vi "Download OD Values.vi"(8 "error in":errorcluster, 10 "Values":T1(array[cluster]) {"Multiplexer"."Index" format="%.0x"}, 11 "Interactor in":refnum<class "Interactor.lvclass">) -> (0 "error out":errorcluster, 3 "Interactor out":refnum<class "Interactor.lvclass">)   [LabVIEW 2024, in "Interactor.lvlib" / "Interactor.lvclass"]
uses:
  Interactor.lvclass
  Interactor.lvclass/Interactor.ctl
  CANopen Master/CANopen Master.lvclass
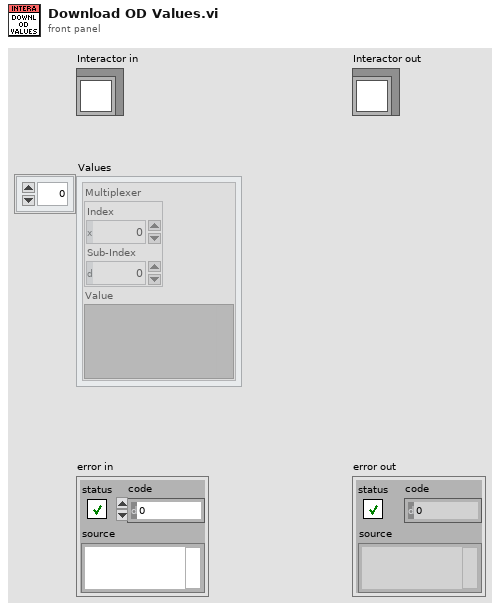
[diagram p1: front panel]
types:
  T1 = cluster{"Multiplexer":cluster{"Index":u16, "Sub-Index":i16}, "Value":variant}[]
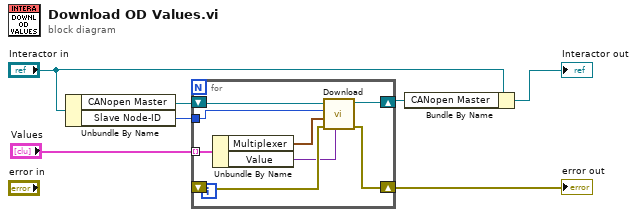
[diagram p0: block diagram]
diagram:
  n1 = Unbundle By Name("Interactor in") -> ("CANopen Master"=w5:refnum<class "CANopen Master.lvclass">, "Slave Node-ID"=w4:u8)
  n2 = for {
    tunnel: "Values" -> [w15] mode=indexing
    shift-right: [w12] -> w6
    shift-left: _ -> [w14]
    tunnel: w4 -> [w9]
    shift-right: [w11] -> w2
    shift-left: w5 -> [w10]
    n3 = Unbundle By Name(w15) -> ("Multiplexer"=w8:cluster{"Index":u16, "Sub-Index":i16}, "Value"=w13:variant)
    n4 = call "Download.vi"("Value"=w13, "error in"=w14, "Multiplexer"=w8, "Node-ID"=w9, "CANopen Master in"=w10) -> ("error out"=w12:errorcluster, "CANopen Master out"=w11:refnum<class "CANopen Master.lvclass">)  [unwired: 4 in, 1 out]
  }
  "error out" <- w6
  n5 = Bundle By Name(cluster="Interactor in", "CANopen Master"=w2) -> (→"Interactor out":refnum<class "Interactor.lvclass">)
